vi "DC Transport Measure.vi"(4 "Channel 2":bool, 5 "Voltmeter 2 Address":string="8", 6 "Channel 1":bool=TRUE, 7 "Voltmeter 1 Address":string="7", 8 "tpad":i32=100, 9 "Period (s)":string="3", 10 "Amplitude (A)":string="1e-4", 11 "6221 Address":string="12") -> (0 "STD 2":dbl=0.00015789614384998, 1 "Resistance 2":dbl=0.023133111600000002, 2 "STD 1":dbl=0.0001111117115108547, 3 "Resistance 1":dbl=3.9215312102230766)   [LabVIEW 2020]
uses:
  <vilib>/Instr/_visa.llb/GPIB Status Boolean Array.ctl
panel:
  out "Buffer 2 Data":dbl[][](array[numeric])=[[0.0, 1.69853343e-06], [0.05, 2.29085744e-06], [0.101, 2.2689427e-06], [0.152, 2.25641999e-06], [0.203, 2.27896086e-06], [0.254, 2.27332565e-06], [0.305, 2.24828023e-06], [0.356, 2.26142908e-06], [0.407, 2.27708246e-06], [0.458, 2.26268135e-06], [0.509, 2.28146541e-06], [0.56, 2.27520405e-06], [0.611, 2.25266318e-06], [0.662, 2.27207338e-06], [0.713, 2.26268135e-06], [0.764, 2.26455975e-06], [0.815, 2.27457792e-06], [0.866, 2.25892453e-06], [0.917, 2.28021313e-06], [0.968, 2.27144724e-06], [1.019, 2.2495325e-06], [1.07, 2.24201888e-06], [1.121, 2.2476541e-06], [1.172, 2.23763593e-06], [1.223, 2.25203705e-06], [1.274, 2.22260869e-06], [1.325, 2.25892453e-06], [1.376, 2.2689427e-06], [1.427, 2.23262685e-06], [1.478, 1.17257976e-06], [1.529, -2.35755925e-06], [1.58, -2.36006378e-06], [1.631, -2.37696934e-06], [1.681, -2.35192407e-06], [1.731, -2.35630699e-06], [1.781, -2.34628888e-06], [1.832, -2.35881152e-06], [1.882, -2.33188785e-06], [1.932, -2.33814917e-06], [1.982, -2.34941954e-06], [2.032, -2.3368969e-06], [2.083, -2.3782216e-06], [2.133, -2.36131604e-06], [2.183, -2.33752304e-06], [2.233, -2.36256831e-06], [2.283, -2.38135226e-06], [2.333, -2.36757736e-06], [2.384, -2.36068991e-06], [2.434, -2.37133415e-06], [2.484, -2.3782216e-06], [2.534, -2.3763432e-06], [2.584, -2.37696934e-06], [2.635, -2.37133415e-06], [2.685, -2.40264074e-06], [2.735, -2.37321255e-06], [2.785, -2.3801e-06], [2.835, -2.37947386e-06], [2.885, -2.38636131e-06], [2.935, -2.36882962e-06], [2.985, -1.36075749e-06], [3.035, -5.33931926e-08], [3.085, -3.6487539e-08]]
  out "Buffer 2 Plot":cluster{dbl[], dbl[]}(graph)={[0.0, 0.05, 0.101, 0.152, 0.203, 0.254, 0.305, 0.356, 0.407, 0.458, 0.509, 0.56, 0.611, 0.662, 0.713, 0.764, 0.815, 0.866, 0.917, 0.968, 1.019, 1.07, 1.121, 1.172, 1.223, 1.274, 1.325, 1.376, 1.427, 1.478, 1.529, 1.58, 1.631, 1.681, 1.731, 1.781, 1.832, 1.882, 1.932, 1.982, 2.032, 2.083, 2.133, 2.183, 2.233, 2.283, 2.333, 2.384, 2.434, 2.484, 2.534, 2.584, 2.635, 2.685, 2.735, 2.785, 2.835, 2.885, 2.935, 2.985, 3.035, 3.085], [1.69853343e-06, 2.29085744e-06, 2.2689427e-06, 2.25641999e-06, 2.27896086e-06, 2.27332565e-06, 2.24828023e-06, 2.26142908e-06, 2.27708246e-06, 2.26268135e-06, 2.28146541e-06, 2.27520405e-06, 2.25266318e-06, 2.27207338e-06, 2.26268135e-06, 2.26455975e-06, 2.27457792e-06, 2.25892453e-06, 2.28021313e-06, 2.27144724e-06, 2.2495325e-06, 2.24201888e-06, 2.2476541e-06, 2.23763593e-06, 2.25203705e-06, 2.22260869e-06, 2.25892453e-06, 2.2689427e-06, 2.23262685e-06, 1.17257976e-06, -2.35755925e-06, -2.36006378e-06, -2.37696934e-06, -2.35192407e-06, -2.35630699e-06, -2.34628888e-06, -2.35881152e-06, -2.33188785e-06, -2.33814917e-06, -2.34941954e-06, -2.3368969e-06, -2.3782216e-06, -2.36131604e-06, -2.33752304e-06, -2.36256831e-06, -2.38135226e-06, -2.36757736e-06, -2.36068991e-06, -2.37133415e-06, -2.3782216e-06, -2.3763432e-06, -2.37696934e-06, -2.37133415e-06, -2.40264074e-06, -2.37321255e-06, -2.3801e-06, -2.37947386e-06, -2.38636131e-06, -2.36882962e-06, -1.36075749e-06, -5.33931926e-08, -3.6487539e-08]}
  out "Voltage 2":dbl[](array[numeric])=[2.31331116e-06, 1.5789614384998e-08]
  out "Python error 2":errorcluster
  out "T2":dbl[](array[numeric])=[0.0, 0.05, 0.101, 0.152, 0.203, 0.254, 0.305, 0.356, 0.407, 0.458, 0.509, 0.56, 0.611, 0.662, 0.713, 0.764, 0.815, 0.866, 0.917, 0.968, 1.019, 1.07, 1.121, 1.172, 1.223, 1.274, 1.325, 1.376, 1.427, 1.478, 1.529, 1.58, 1.631, 1.681, 1.731, 1.781, 1.832, 1.882, 1.932, 1.982, 2.032, 2.083, 2.133, 2.183, 2.233, 2.283, 2.333, 2.384, 2.434, 2.484, 2.534, 2.584, 2.635, 2.685, 2.735, 2.785, 2.835, 2.885, 2.935, 2.985, 3.035, 3.085]
  out "V2":dbl[](array[numeric])=[1.69853343e-06, 2.29085744e-06, 2.2689427e-06, 2.25641999e-06, 2.27896086e-06, 2.27332565e-06, 2.24828023e-06, 2.26142908e-06, 2.27708246e-06, 2.26268135e-06, 2.28146541e-06, 2.27520405e-06, 2.25266318e-06, 2.27207338e-06, 2.26268135e-06, 2.26455975e-06, 2.27457792e-06, 2.25892453e-06, 2.28021313e-06, 2.27144724e-06, 2.2495325e-06, 2.24201888e-06, 2.2476541e-06, 2.23763593e-06, 2.25203705e-06, 2.22260869e-06, 2.25892453e-06, 2.2689427e-06, 2.23262685e-06, 1.17257976e-06, -2.35755925e-06, -2.36006378e-06, -2.37696934e-06, -2.35192407e-06, -2.35630699e-06, -2.34628888e-06, -2.35881152e-06, -2.33188785e-06, -2.33814917e-06, -2.34941954e-06, -2.3368969e-06, -2.3782216e-06, -2.36131604e-06, -2.33752304e-06, -2.36256831e-06, -2.38135226e-06, -2.36757736e-06, -2.36068991e-06, -2.37133415e-06, -2.3782216e-06, -2.3763432e-06, -2.37696934e-06, -2.37133415e-06, -2.40264074e-06, -2.37321255e-06, -2.3801e-06, -2.37947386e-06, -2.38636131e-06, -2.36882962e-06, -1.36075749e-06, -5.33931926e-08, -3.6487539e-08]
  out "Write Status 2":T1=[FALSE, FALSE, FALSE, FALSE, FALSE, FALSE, FALSE, FALSE, TRUE, FALSE, FALSE, FALSE, FALSE, FALSE, FALSE, FALSE]
  out "error out 2":errorcluster
  out "Read Status 2":T1=[FALSE, FALSE, FALSE, FALSE, FALSE, FALSE, FALSE, FALSE, TRUE, FALSE, FALSE, FALSE, FALSE, TRUE, FALSE, FALSE]
  out "Buffer 1 Data":dbl[][](array[numeric])=[[0.0, 0.00036749345], [0.05, 0.000410422176], [0.1, 0.000410440316], [0.15, 0.000410443444], [0.201, 0.000410440316], [0.251, 0.000410435312], [0.301, 0.000410462209], [0.351, 0.000410434061], [0.401, 0.000410437814], [0.451, 0.000410449699], [0.501, 0.000410454077], [0.552, 0.000410440316], [0.602, 0.000410456579], [0.652, 0.000410457205], [0.702, 0.000410462209], [0.753, 0.000410470966], [0.803, 0.000410467839], [0.853, 0.000410449699], [0.903, 0.000410437814], [0.953, 0.000410442193], [1.003, 0.000410455954], [1.053, 0.00041046909], [1.103, 0.000410447197], [1.154, 0.000410452201], [1.204, 0.000410461583], [1.254, 0.000410442818], [1.304, 0.000410466588], [1.354, 0.000410446571], [1.404, 0.000410449699], [1.454, 0.000410474719], [1.505, -0.000362004013], [1.554, -0.000373841107], [1.605, -0.000373848613], [1.655, -0.000373849864], [1.704, -0.000373856119], [1.755, -0.000373844234], [1.805, -0.00037385174], [1.855, -0.000373866127], [1.904, -0.000373854868], [1.955, -0.00037386988], [2.005, -0.000373834852], [2.054, -0.000373862999], [2.105, -0.000373861123], [2.155, -0.000373840481], [2.204, -0.00037385737], [2.254, -0.00037386988], [2.305, -0.000373842358], [2.355, -0.000373854242], [2.404, -0.000373844234], [2.455, -0.000373861123], [2.505, -0.000373859246], [2.555, -0.000373862374], [2.604, -0.000373846111], [2.655, -0.000373831724], [2.705, -0.00037386425], [2.754, -0.000373862374], [2.805, -0.00037385174], [2.855, -0.000373879263], [2.905, -0.000373831724], [2.954, -0.000373857995], [3.005, 1.82924358e-05], [3.055, 1.82818021e-05], [3.106, 1.82774235e-05], [3.106, 1.82774235e-05], [3.106, 1.82774235e-05], [3.106, 1.82774235e-05], [3.106, 1.82774235e-05], [3.106, 1.82774235e-05], [3.106, 1.82774235e-05], [3.106, 1.82774235e-05], [3.106, 1.82774235e-05], [3.106, 1.82774235e-05], [3.106, 1.82774235e-05], [3.106, 1.82774235e-05], [3.106, 1.82774235e-05], [3.106, 1.82774235e-05], [3.106, 1.82774235e-05], [3.106, 1.82774235e-05], [3.106, 1.82774235e-05], [3.106, 1.82774235e-05], [3.106, 1.82774235e-05], [3.106, 1.82774235e-05]]
  out "Buffer 1 Plot":cluster{dbl[], dbl[]}(graph)={[0.0, 0.05, 0.1, 0.15, 0.201, 0.251, 0.301, 0.351, 0.401, 0.451, 0.501, 0.552, 0.602, 0.652, 0.702, 0.753, 0.803, 0.853, 0.903, 0.953, 1.003, 1.053, 1.103, 1.154, 1.204, 1.254, 1.304, 1.354, 1.404, 1.454, 1.505, 1.554, 1.605, 1.655, 1.704, 1.755, 1.805, 1.855, 1.904, 1.955, 2.005, 2.054, 2.105, 2.155, 2.204, 2.254, 2.305, 2.355, 2.404, 2.455, 2.505, 2.555, 2.604, 2.655, 2.705, 2.754, 2.805, 2.855, 2.905, 2.954, 3.005, 3.055, 3.106, 3.106, 3.106, 3.106, 3.106, 3.106, 3.106, 3.106, 3.106, 3.106, 3.106, 3.106, 3.106, 3.106, 3.106, 3.106, 3.106, 3.106, 3.106, 3.106], [0.00036749345, 0.000410422176, 0.000410440316, 0.000410443444, 0.000410440316, 0.000410435312, 0.000410462209, 0.000410434061, 0.000410437814, 0.000410449699, 0.000410454077, 0.000410440316, 0.000410456579, 0.000410457205, 0.000410462209, 0.000410470966, 0.000410467839, 0.000410449699, 0.000410437814, 0.000410442193, 0.000410455954, 0.00041046909, 0.000410447197, 0.000410452201, 0.000410461583, 0.000410442818, 0.000410466588, 0.000410446571, 0.000410449699, 0.000410474719, -0.000362004013, -0.000373841107, -0.000373848613, -0.000373849864, -0.000373856119, -0.000373844234, -0.00037385174, -0.000373866127, -0.000373854868, -0.00037386988, -0.000373834852, -0.000373862999, -0.000373861123, -0.000373840481, -0.00037385737, -0.00037386988, -0.000373842358, -0.000373854242, -0.000373844234, -0.000373861123, -0.000373859246, -0.000373862374, -0.000373846111, -0.000373831724, -0.00037386425, -0.000373862374, -0.00037385174, -0.000373879263, -0.000373831724, -0.000373857995, 1.82924358e-05, 1.82818021e-05, 1.82774235e-05, 1.82774235e-05, 1.82774235e-05, 1.82774235e-05, 1.82774235e-05, 1.82774235e-05, 1.82774235e-05, 1.82774235e-05, 1.82774235e-05, 1.82774235e-05, 1.82774235e-05, 1.82774235e-05, 1.82774235e-05, 1.82774235e-05, 1.82774235e-05, 1.82774235e-05, 1.82774235e-05, 1.82774235e-05, 1.82774235e-05, 1.82774235e-05]}
  in  "Python Support File":path=path "C:/Users/QDUser/Desktop/LabVIEW Programs/PPMS Interface/lib/PPMS External Control Support.py"
  out "Voltage 1":dbl[](array[numeric])=[0.0003921531210223077, 1.111117115108547e-08]
  out "Python error":errorcluster
  out "T1":dbl[](array[numeric])=[0.0, 0.05, 0.1, 0.15, 0.201, 0.251, 0.301, 0.351, 0.401, 0.451, 0.501, 0.552, 0.602, 0.652, 0.702, 0.753, 0.803, 0.853, 0.903, 0.953, 1.003, 1.053, 1.103, 1.154, 1.204, 1.254, 1.304, 1.354, 1.404, 1.454, 1.505, 1.554, 1.605, 1.655, 1.704, 1.755, 1.805, 1.855, 1.904, 1.955, 2.005, 2.054, 2.105, 2.155, 2.204, 2.254, 2.305, 2.355, 2.404, 2.455, 2.505, 2.555, 2.604, 2.655, 2.705, 2.754, 2.805, 2.855, 2.905, 2.954, 3.005, 3.055, 3.106, 3.106, 3.106, 3.106, 3.106, 3.106, 3.106, 3.106, 3.106, 3.106, 3.106, 3.106, 3.106, 3.106, 3.106, 3.106, 3.106, 3.106, 3.106, 3.106]
  out "V1":dbl[](array[numeric])=[0.00036749345, 0.000410422176, 0.000410440316, 0.000410443444, 0.000410440316, 0.000410435312, 0.000410462209, 0.000410434061, 0.000410437814, 0.000410449699, 0.000410454077, 0.000410440316, 0.000410456579, 0.000410457205, 0.000410462209, 0.000410470966, 0.000410467839, 0.000410449699, 0.000410437814, 0.000410442193, 0.000410455954, 0.00041046909, 0.000410447197, 0.000410452201, 0.000410461583, 0.000410442818, 0.000410466588, 0.000410446571, 0.000410449699, 0.000410474719, -0.000362004013, -0.000373841107, -0.000373848613, -0.000373849864, -0.000373856119, -0.000373844234, -0.00037385174, -0.000373866127, -0.000373854868, -0.00037386988, -0.000373834852, -0.000373862999, -0.000373861123, -0.000373840481, -0.00037385737, -0.00037386988, -0.000373842358, -0.000373854242, -0.000373844234, -0.000373861123, -0.000373859246, -0.000373862374, -0.000373846111, -0.000373831724, -0.00037386425, -0.000373862374, -0.00037385174, -0.000373879263, -0.000373831724, -0.000373857995, 1.82924358e-05, 1.82818021e-05, 1.82774235e-05, 1.82774235e-05, 1.82774235e-05, 1.82774235e-05, 1.82774235e-05, 1.82774235e-05, 1.82774235e-05, 1.82774235e-05, 1.82774235e-05, 1.82774235e-05, 1.82774235e-05, 1.82774235e-05, 1.82774235e-05, 1.82774235e-05, 1.82774235e-05, 1.82774235e-05, 1.82774235e-05, 1.82774235e-05, 1.82774235e-05, 1.82774235e-05]
  out "Write Status":T1=[FALSE, FALSE, FALSE, FALSE, FALSE, FALSE, FALSE, FALSE, TRUE, FALSE, FALSE, FALSE, FALSE, FALSE, FALSE, FALSE]
  in  "Byte Count":i32=2000
  out "error out":errorcluster
  out "Read Status":T1=[FALSE, FALSE, FALSE, FALSE, FALSE, FALSE, FALSE, FALSE, TRUE, FALSE, FALSE, FALSE, FALSE, TRUE, FALSE, FALSE]
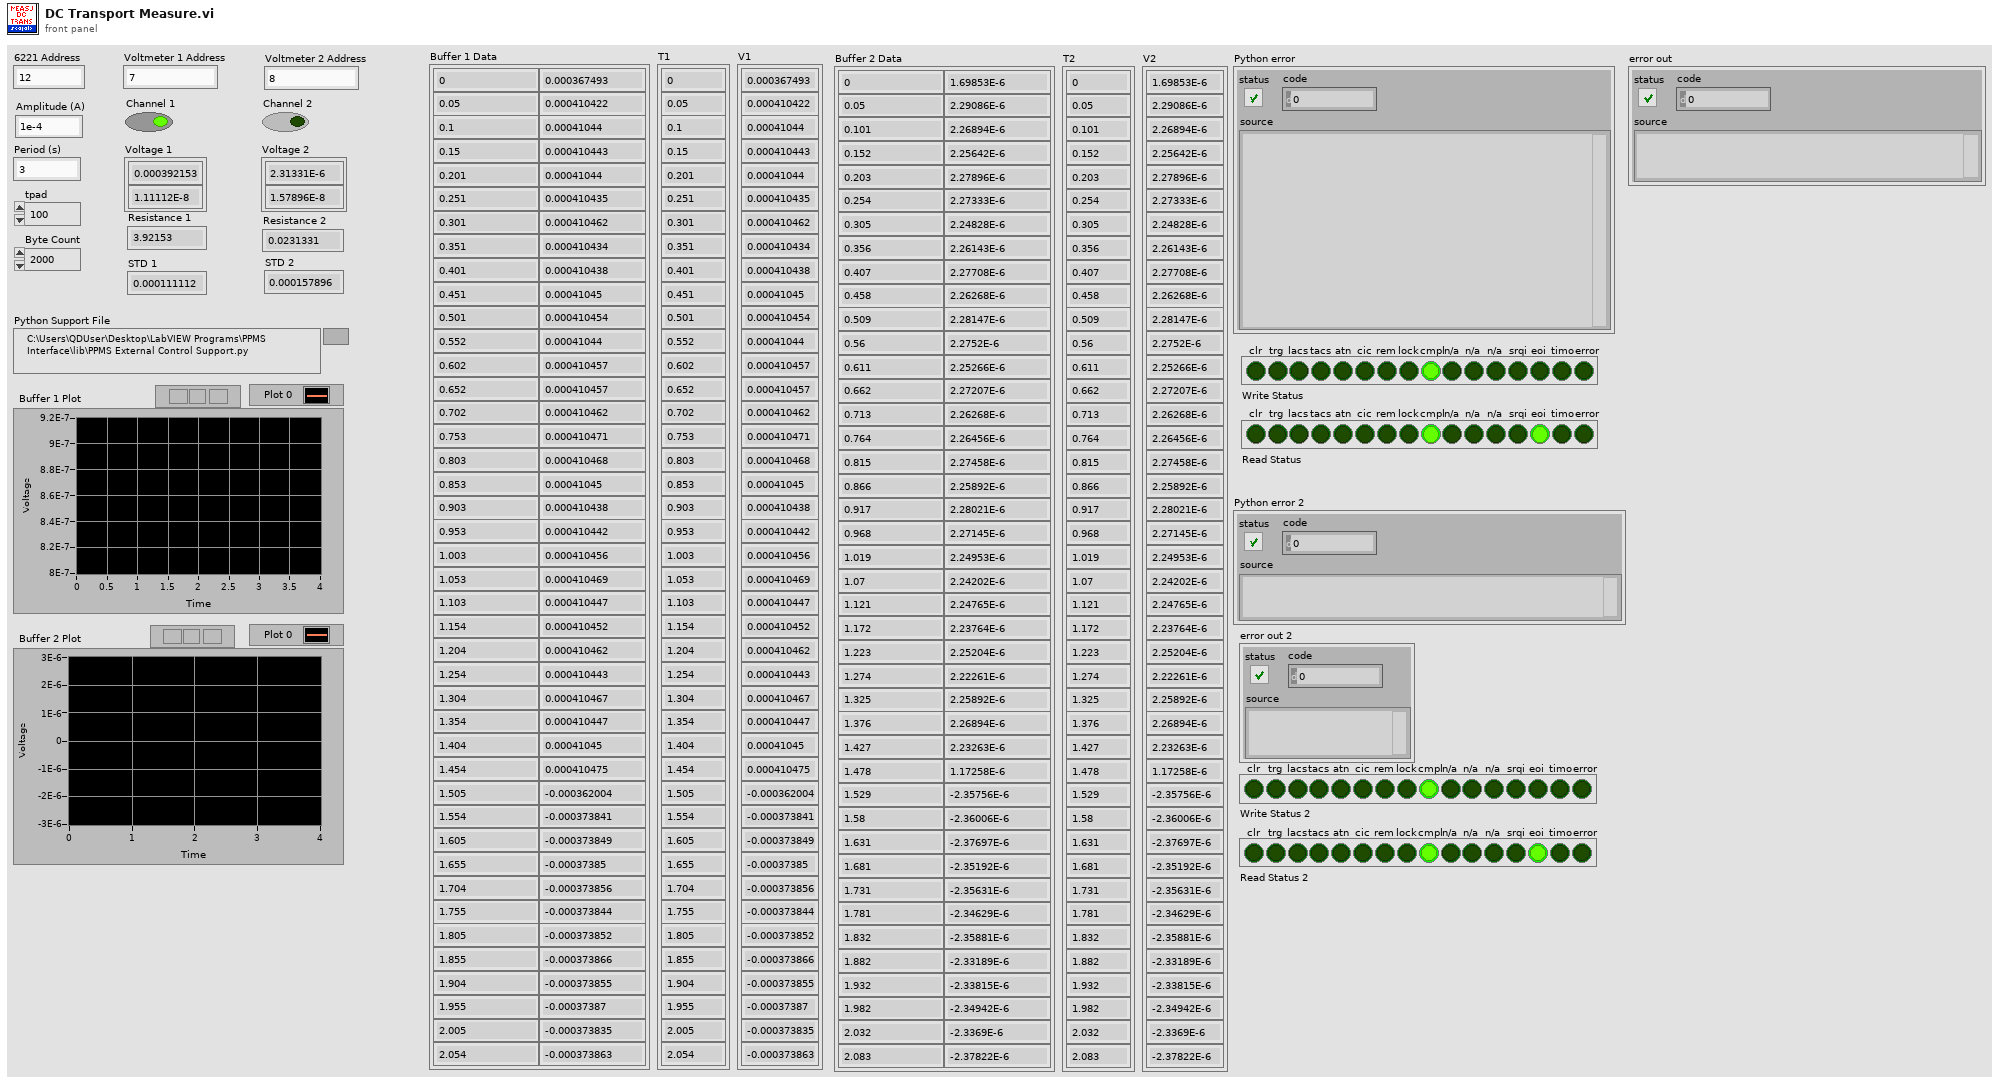
[diagram p1: front panel]
types:
  T1 = typedef "GPIB Status Boolean Array.ctl" = bool[]
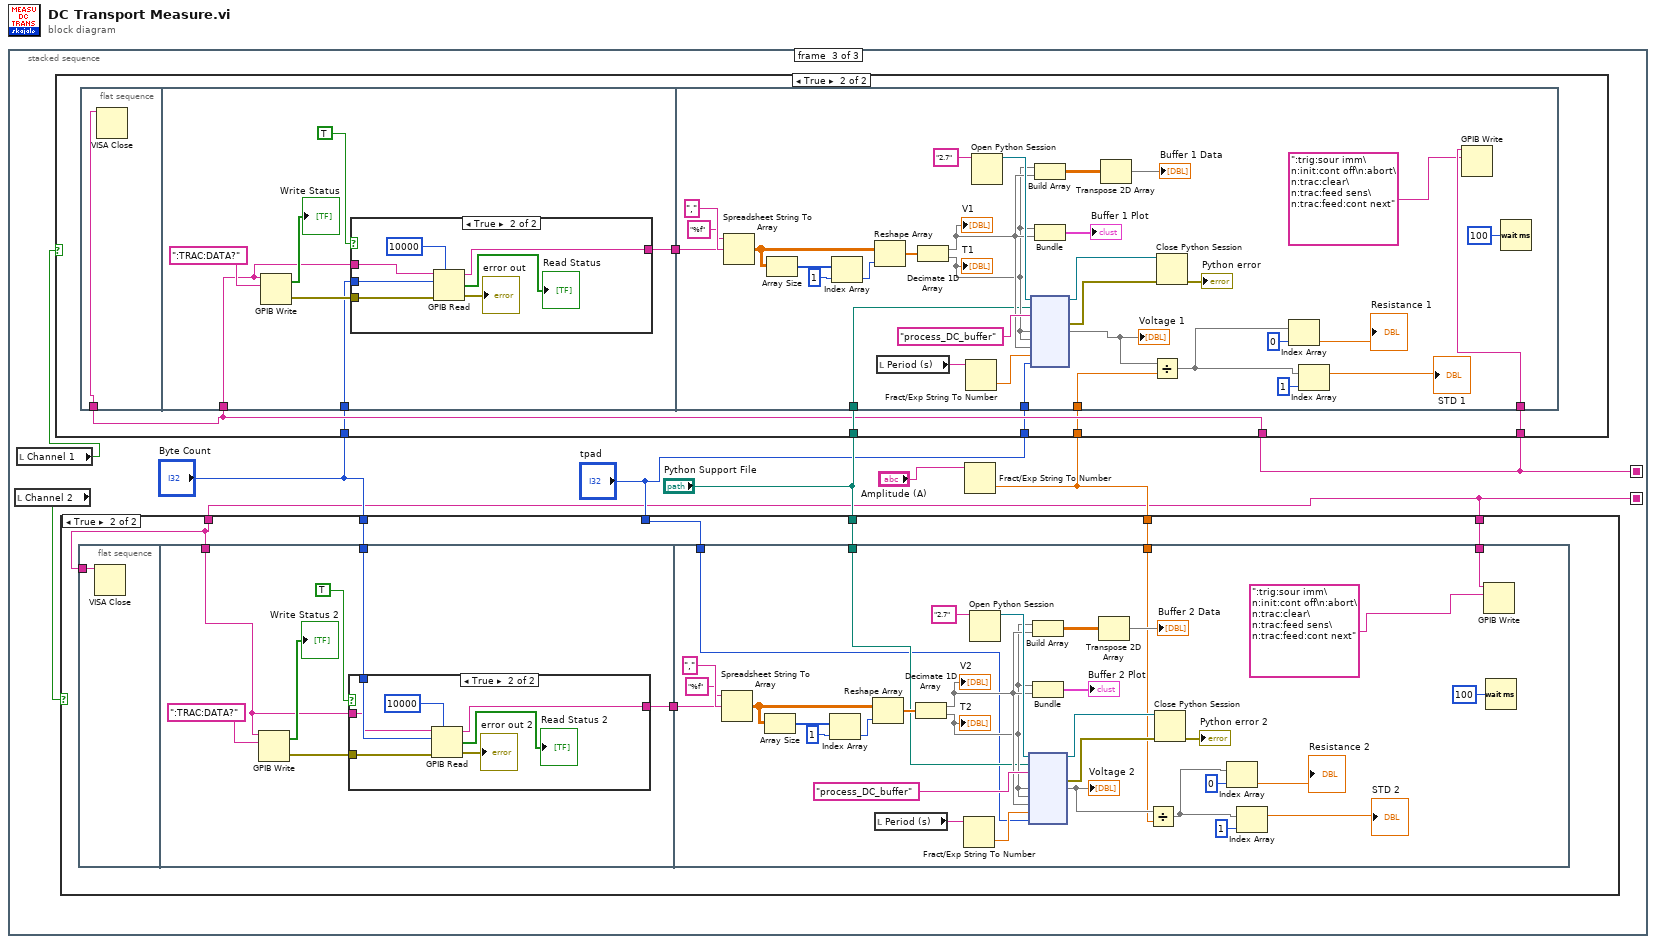
[diagram p0: block diagram]
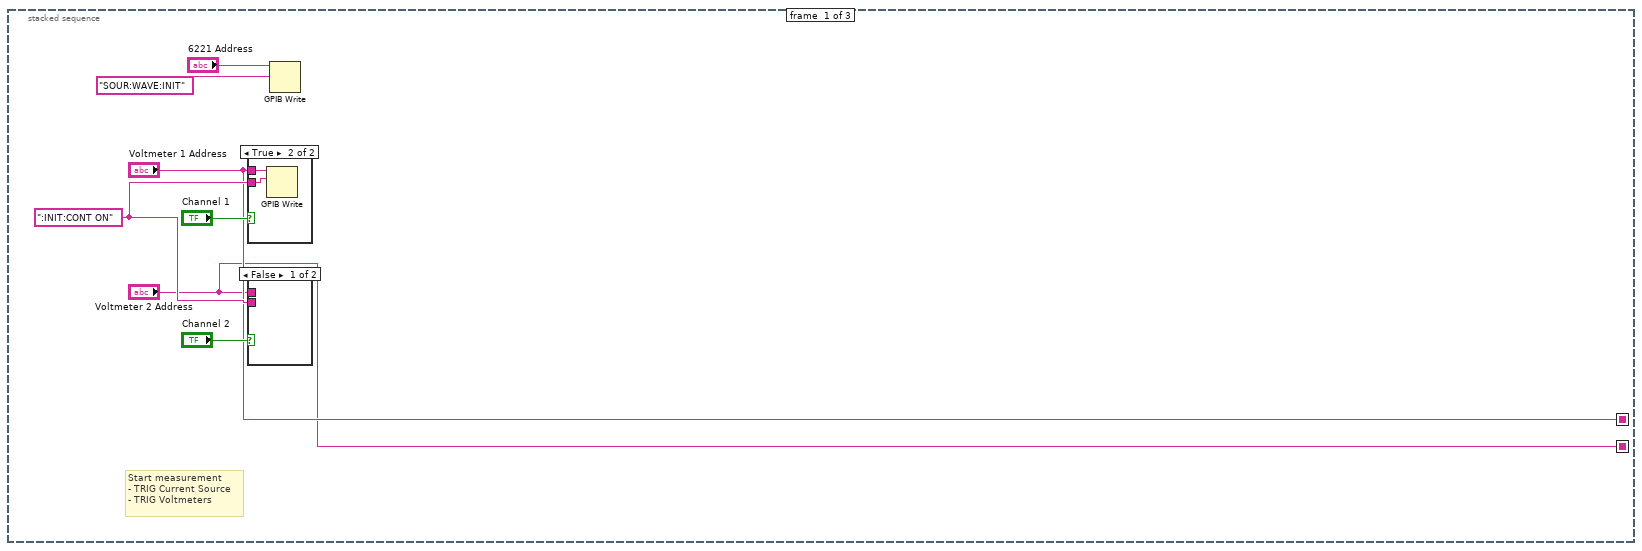
[diagram p2: hidden frame]
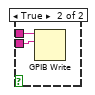
[diagram p4: hidden frame]
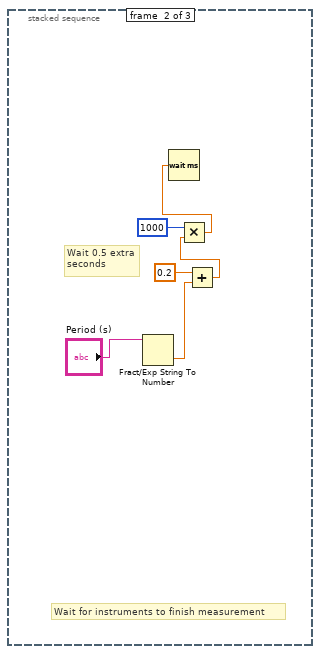
[diagram p5: hidden frame]
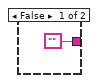
[diagram p7: hidden frame]
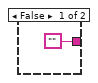
[diagram p9: hidden frame]
diagram:
  n1 = stacked-sequence {
    seq-local: ["Voltmeter 1 Address" _ _] -> [_ _ w19]
    seq-local: ["Voltmeter 2 Address" _ _] -> [_ _ w18]
    frame #0 {
      w3 = ":INIT:CONT ON" ("data")
      # "Start measurement\n- TRIG Current Source\n- TRIG Voltmeters"
      n2 = case shown="True" "Channel 1" {
        tunnel: "Voltmeter 1 Address" -> [_ w9]
        tunnel: w3 -> [_ w8]
        frame False {
        }
        frame True {
          n3 = GPIB Write(0:w9, 1:w8) -> ()  [unwired: 3 in, 2 out]
        }
      }
      n4 = case shown="False" "Channel 2" {
        tunnel: "Voltmeter 2 Address" -> [_ w11]
        tunnel: w3 -> [_ w10]
        frame False {
        }
        frame True {
          n5 = GPIB Write(0:w11, 1:w10) -> ()  [unwired: 3 in, 2 out]
        }
      }
      n6 = GPIB Write(0:"6221 Address", 1:"SOUR:WAVE:INIT" ("data")) -> ()  [unwired: 3 in, 2 out]
    }
    frame #1 {
      # "Wait for instruments to finish measurement"
      # "Wait 0.5 extra\nseconds"
      n7 = Fract/Exp String To Number(string="Period (s)") -> (number=w12:dbl)  [unwired: 3 in, 1 out]
      n8 = Add(x=0.2, y=w12) -> (x+y=w16:dbl)
      n9 = Multiply(x=1000, y=w16) -> (x*y=w14:dbl)
      n10 = Wait (ms)(milliseconds to wait=w14) -> ()  [unwired: 1 out]
    }
    frame #2 {
      n11 = local read "Channel 2"() -> (w25:bool)
      n12 = local read "Channel 1"() -> (w24:bool)
      n13 = Fract/Exp String To Number(string="Amplitude (A)") -> (number=w21:dbl)  [unwired: 3 in, 1 out]
      n14 = case shown="True" w24 {
        tunnel: "Python Support File" -> [_ w88]
        tunnel: w19 -> [_ w87]
        tunnel: "Byte Count" -> [_ w86]
        tunnel: w21 -> [_ w85]
        tunnel: "tpad" -> [_ w84]
        tunnel: w19 -> [_ w83]
        frame False {
        }
        frame True {
          n15 = flat-sequence {
            tunnel: w87 -> [w90]
            tunnel: [w93] -> w89
            tunnel: w87 -> [w91]
            tunnel: w86 -> [w92]
            tunnel: w89 -> [w120]
            tunnel: w88 -> [w117]
            tunnel: w85 -> [w115]
            tunnel: w84 -> [w109]
            tunnel: w83 -> [w108]
            frame #0 {
              n16 = VISA Close(VISA resource name=w90) -> ()  [unwired: 1 in, 1 out]
            }
            frame #1 {
              n17 = GPIB Write(0:w91, 1:":TRAC:DATA?" ("data")) -> (5:→"Write Status":bool[], 6:w96:errorcluster)  [unwired: 3 in]
              n18 = case shown="True" TRUE ("Query?") {
                tunnel: w96 -> [_ w104]
                tunnel: w92 -> [_ w101]
                tunnel: ["" w100] -> w93
                tunnel: w91 -> [_ w99]
                frame False {
                }
                frame True {
                  n19 = GPIB Read(0:w99, 1:w101, 3:w104, 4:10000 ("timeout ms (488.2 global)")) -> (5:w100:string, 6:→"Read Status":bool[], 7:→"error out":errorcluster)  [unwired: 1 in]
                }
              }
            }
            frame #2 {
              n20 = Spreadsheet String To Array(delimiter (Tab)=",", format string="%f", spreadsheet string=w120) -> (array=w137:dbl[][])  [unwired: 1 in]
              n21 = Array Size(array=w137) -> (size(s)=w136:i32[])
              n22 = Index Array(array=w136, index=1) -> (element=w134:i32)
              n23 = Reshape Array(w137, w134) -> (w133:dbl[])
              n24 = local read "Period (s)"() -> (w119:string)
              n25 = Decimate 1D Array(w133) -> (w126:dbl[], w123:dbl[])
              "T1" <- w123
              "V1" <- w126
              n26 = Fract/Exp String To Number(string=w119) -> (number=w118:dbl)  [unwired: 3 in, 1 out]
              n27 = Open Python Session(python version="2.7" ("Python version")) -> (session out=w128:refnum<k35>)  [unwired: 2 in, 1 out]
              n28 = node(w128, w117, "process_DC_buffer" ("Buffer Process Function"), w123, w123, w126, w118, w109) -> (w125:refnum<k35>, w122:errorcluster, w116:dbl[])  [unwired: 5 in, 2 out]
              "Voltage 1" <- w116
              n29 = Build Array(w123, w126) -> (w132:dbl[][])
              n30 = Bundle(w123, w126) -> (→"Buffer 1 Plot":cluster{dbl[], dbl[]})  [unwired: 1 in]
              n31 = Transpose 2D Array(2D array=w132) -> (transposed array=→"Buffer 1 Data":dbl[][])
              n32 = Divide(x=w116, y=w115) -> (x/y=w112:dbl[])
              n33 = Close Python Session(session in=w125, error in=w122) -> (11:→"Python error":errorcluster)
              n34 = Index Array(array=w112, index=0) -> (element=→"Resistance 1":dbl)
              n35 = Index Array(array=w112, index=1) -> (element=→"STD 1":dbl)
              n36 = GPIB Write(0:w108, 1:":trig:sour imm\n:init:cont off\n:abort\n:trac:clear\n:trac:feed sens\n:trac:feed:cont next" ("data")) -> ()  [unwired: 3 in, 2 out]
              n37 = Wait (ms)(milliseconds to wait=u32 100) -> ()  [unwired: 1 out]
            }
          }
        }
      }
      n38 = case shown="True" w25 {
        tunnel: "Python Support File" -> [_ w32]
        tunnel: w18 -> [_ w31]
        tunnel: "Byte Count" -> [_ w30]
        tunnel: w21 -> [_ w29]
        tunnel: "tpad" -> [_ w28]
        tunnel: w18 -> [_ w27]
        frame False {
        }
        frame True {
          n39 = flat-sequence {
            tunnel: w31 -> [w34]
            tunnel: [w37] -> w33
            tunnel: w31 -> [w35]
            tunnel: w30 -> [w36]
            tunnel: w33 -> [w64]
            tunnel: w32 -> [w61]
            tunnel: w29 -> [w59]
            tunnel: w28 -> [w53]
            tunnel: w27 -> [w52]
            frame #0 {
              n40 = VISA Close(VISA resource name=w34) -> ()  [unwired: 1 in, 1 out]
            }
            frame #1 {
              n41 = GPIB Write(0:w35, 1:":TRAC:DATA?" ("data")) -> (5:→"Write Status 2":bool[], 6:w40:errorcluster)  [unwired: 3 in]
              n42 = case shown="True" TRUE ("Query?") {
                tunnel: w40 -> [_ w48]
                tunnel: ["" w45] -> w37
                tunnel: w36 -> [_ w44]
                tunnel: w35 -> [_ w43]
                frame False {
                }
                frame True {
                  n43 = GPIB Read(0:w43, 1:w44, 3:w48, 4:10000 ("timeout ms (488.2 global)")) -> (5:w45:string, 6:→"Read Status 2":bool[], 7:→"error out 2":errorcluster)  [unwired: 1 in]
                }
              }
            }
            frame #2 {
              n44 = Spreadsheet String To Array(delimiter (Tab)=",", format string="%f", spreadsheet string=w64) -> (array=w81:dbl[][])  [unwired: 1 in]
              n45 = Array Size(array=w81) -> (size(s)=w80:i32[])
              n46 = Index Array(array=w80, index=1) -> (element=w78:i32)
              n47 = Reshape Array(w81, w78) -> (w77:dbl[])
              n48 = local read "Period (s)"() -> (w63:string)
              n49 = Decimate 1D Array(w77) -> (w70:dbl[], w67:dbl[])
              "T2" <- w67
              "V2" <- w70
              n50 = Fract/Exp String To Number(string=w63) -> (number=w62:dbl)  [unwired: 3 in, 1 out]
              n51 = Open Python Session(python version="2.7" ("Python version")) -> (session out=w72:refnum<k35>)  [unwired: 2 in, 1 out]
              n52 = node(w72, w61, "process_DC_buffer" ("Buffer Process Function"), w67, w67, w70, w62, w53) -> (w69:refnum<k35>, w66:errorcluster, w60:dbl[])  [unwired: 5 in, 2 out]
              "Voltage 2" <- w60
              n53 = Build Array(w67, w70) -> (w76:dbl[][])
              n54 = Bundle(w67, w70) -> (→"Buffer 2 Plot":cluster{dbl[], dbl[]})  [unwired: 1 in]
              n55 = Transpose 2D Array(2D array=w76) -> (transposed array=→"Buffer 2 Data":dbl[][])
              n56 = Divide(x=w60, y=w59) -> (x/y=w54:dbl[])
              n57 = Close Python Session(session in=w69, error in=w66) -> (11:→"Python error 2":errorcluster)
              n58 = Index Array(array=w54, index=0) -> (element=→"Resistance 2":dbl)
              n59 = Index Array(array=w54, index=1) -> (element=→"STD 2":dbl)
              n60 = GPIB Write(0:w52, 1:":trig:sour imm\n:init:cont off\n:abort\n:trac:clear\n:trac:feed sens\n:trac:feed:cont next" ("data")) -> ()  [unwired: 3 in, 2 out]
              n61 = Wait (ms)(milliseconds to wait=u32 100) -> ()  [unwired: 1 out]
            }
          }
        }
      }
    }
  }
